vi "GetLowProcessAlarmLimit.vi"(8 "error in":errorcluster, 10 "Channel Number (1-4)":T1=1 items=["Channel 1"=1, "Channel 2"=2, "Channel 3"=3, "Channel 4"=4], 11 "VISA resource name":refnum<visa-resource-name>) -> (0 "error out":errorcluster, 2 "Low process alarm limit":string, 3 "VISA resource name out":refnum<visa-resource-name>)   [LabVIEW 2023, in "Thermotron 8800.lvlib"]
doc: "PALL\nCommand name: Send low process alarm limit\nCommand type: Program status\nDescription: Queries the 8800 for a channel’s low process alarm limit. The 8800 sends an integer indicating the alarm limit.\nSyntax: PALLn?\nWhere n is a channel number.\nData type: Integer\nQuery example: PALL1?\n8800 response: -40 (The channel 1 low process alarm limit is -40.)"
uses:
  Thermotron 8800.lvlib
  Private/AnalogInputChannelNumber 1-4.ctl
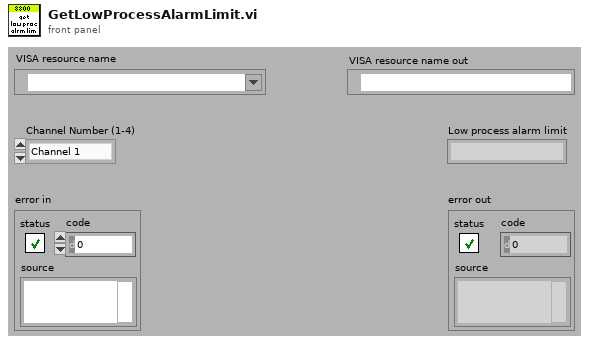
[diagram p1: front panel]
types:
  T1 = typedef "Thermotron 8800.lvlib/AnalogInputChannelNumber 1-4.ctl" = u16
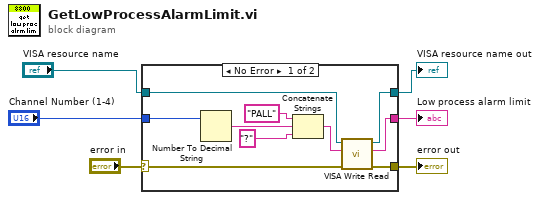
[diagram p0: block diagram]
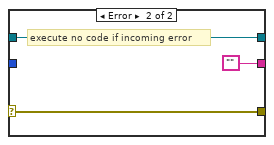
[diagram p2: hidden frame]
diagram:
  n1 = case shown="No Error" "error in" {
    selector: "error in" -> [w14 w18]
    tunnel: [w11 w18] -> w5
    tunnel: [w12 w19] -> w4
    tunnel: "VISA resource name" -> [w13 w19]
    tunnel: [w10 ""] -> w2
    tunnel: "Channel Number (1-4)" -> [w7 _]
    frame No Error {
      n2 = Number To Decimal String(number=w7) -> (decimal integer string=w8:string)  [unwired: 1 in]
      n3 = Concatenate Strings("PALL" ("8800 Command"), w8, "?" ("8800 Command")) -> (w16:string)
      n4 = call "VISA Write Read.vi"("error in (no error)"=w14, "8800 Command"=w16, "VISA Refnum in"=w13) -> ("error out"=w11:errorcluster, "read buffer"=w10:string, "VISA Refnum out"=w12:refnum<visa-resource-name>)  [unwired: 6 in]
    }
    frame Error {
      # "execute no code if incoming error"
    }
  }
  "VISA resource name out" <- w4
  "error out" <- w5
  "Low process alarm limit" <- w2
